vi "Read Boolean.vi"(8 "error in":errorcluster, 10 "register offset":u32, 11 "session in":u32) -> (0 "error out":errorcluster, 2 "value out":bool, 3 "session out":u32)   [LabVIEW 2018, in "Scalar IO Operations.lvlib"]
uses:
  Scalar IO Operations.lvlib
  NiFpga.dll
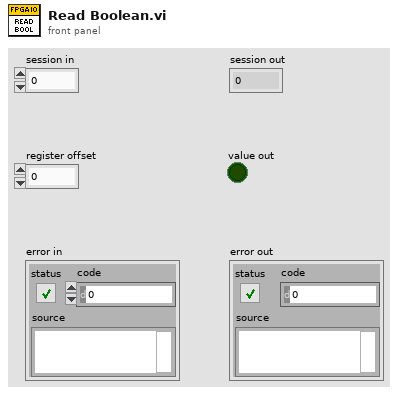
[diagram p1: front panel]
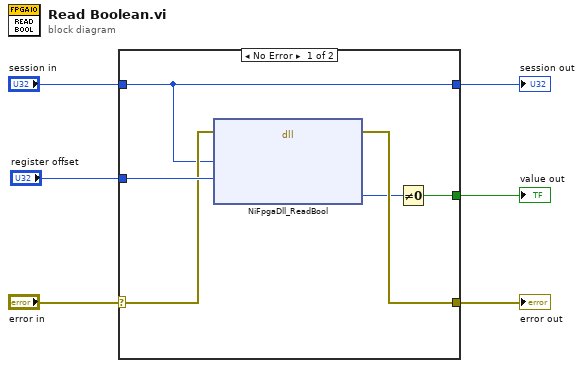
[diagram p0: block diagram]
diagram:
  n1 = case shown="No Error" "error in" {
    selector: "error in" -> [w10 w14]
    tunnel: "session in" -> [w9 w13]
    tunnel: [w12 w14] -> w5
    tunnel: [w8 _] -> w1
    tunnel: "register offset" -> [w11 _]
    tunnel: [w9 w13] -> w2
    frame No Error {
      n2 = dll-call lib="NiFpga.*" fn="NiFpgaDll_ReadBool"(error in=w10, "session"=w9, "offset"=w11) -> (error out=w12:errorcluster, "value"=w7:u8)  [unwired: 6 in, 1 out]
      n3 = Not Equal To 0?(x=w7) -> (x != 0?=w8:bool)
    }
    frame Error {
    }
  }
  "error out" <- w5
  "session out" <- w2
  "value out" <- w1
